vi "ReadnanoVNA.vi"() -> ()   [LabVIEW 2020]
panel:
  out "nanoVNA APP":T1
  out "string array 2":string[][](array[string])
  out "string array":string[](array[string])
  out "after substring":string
  out "text":string
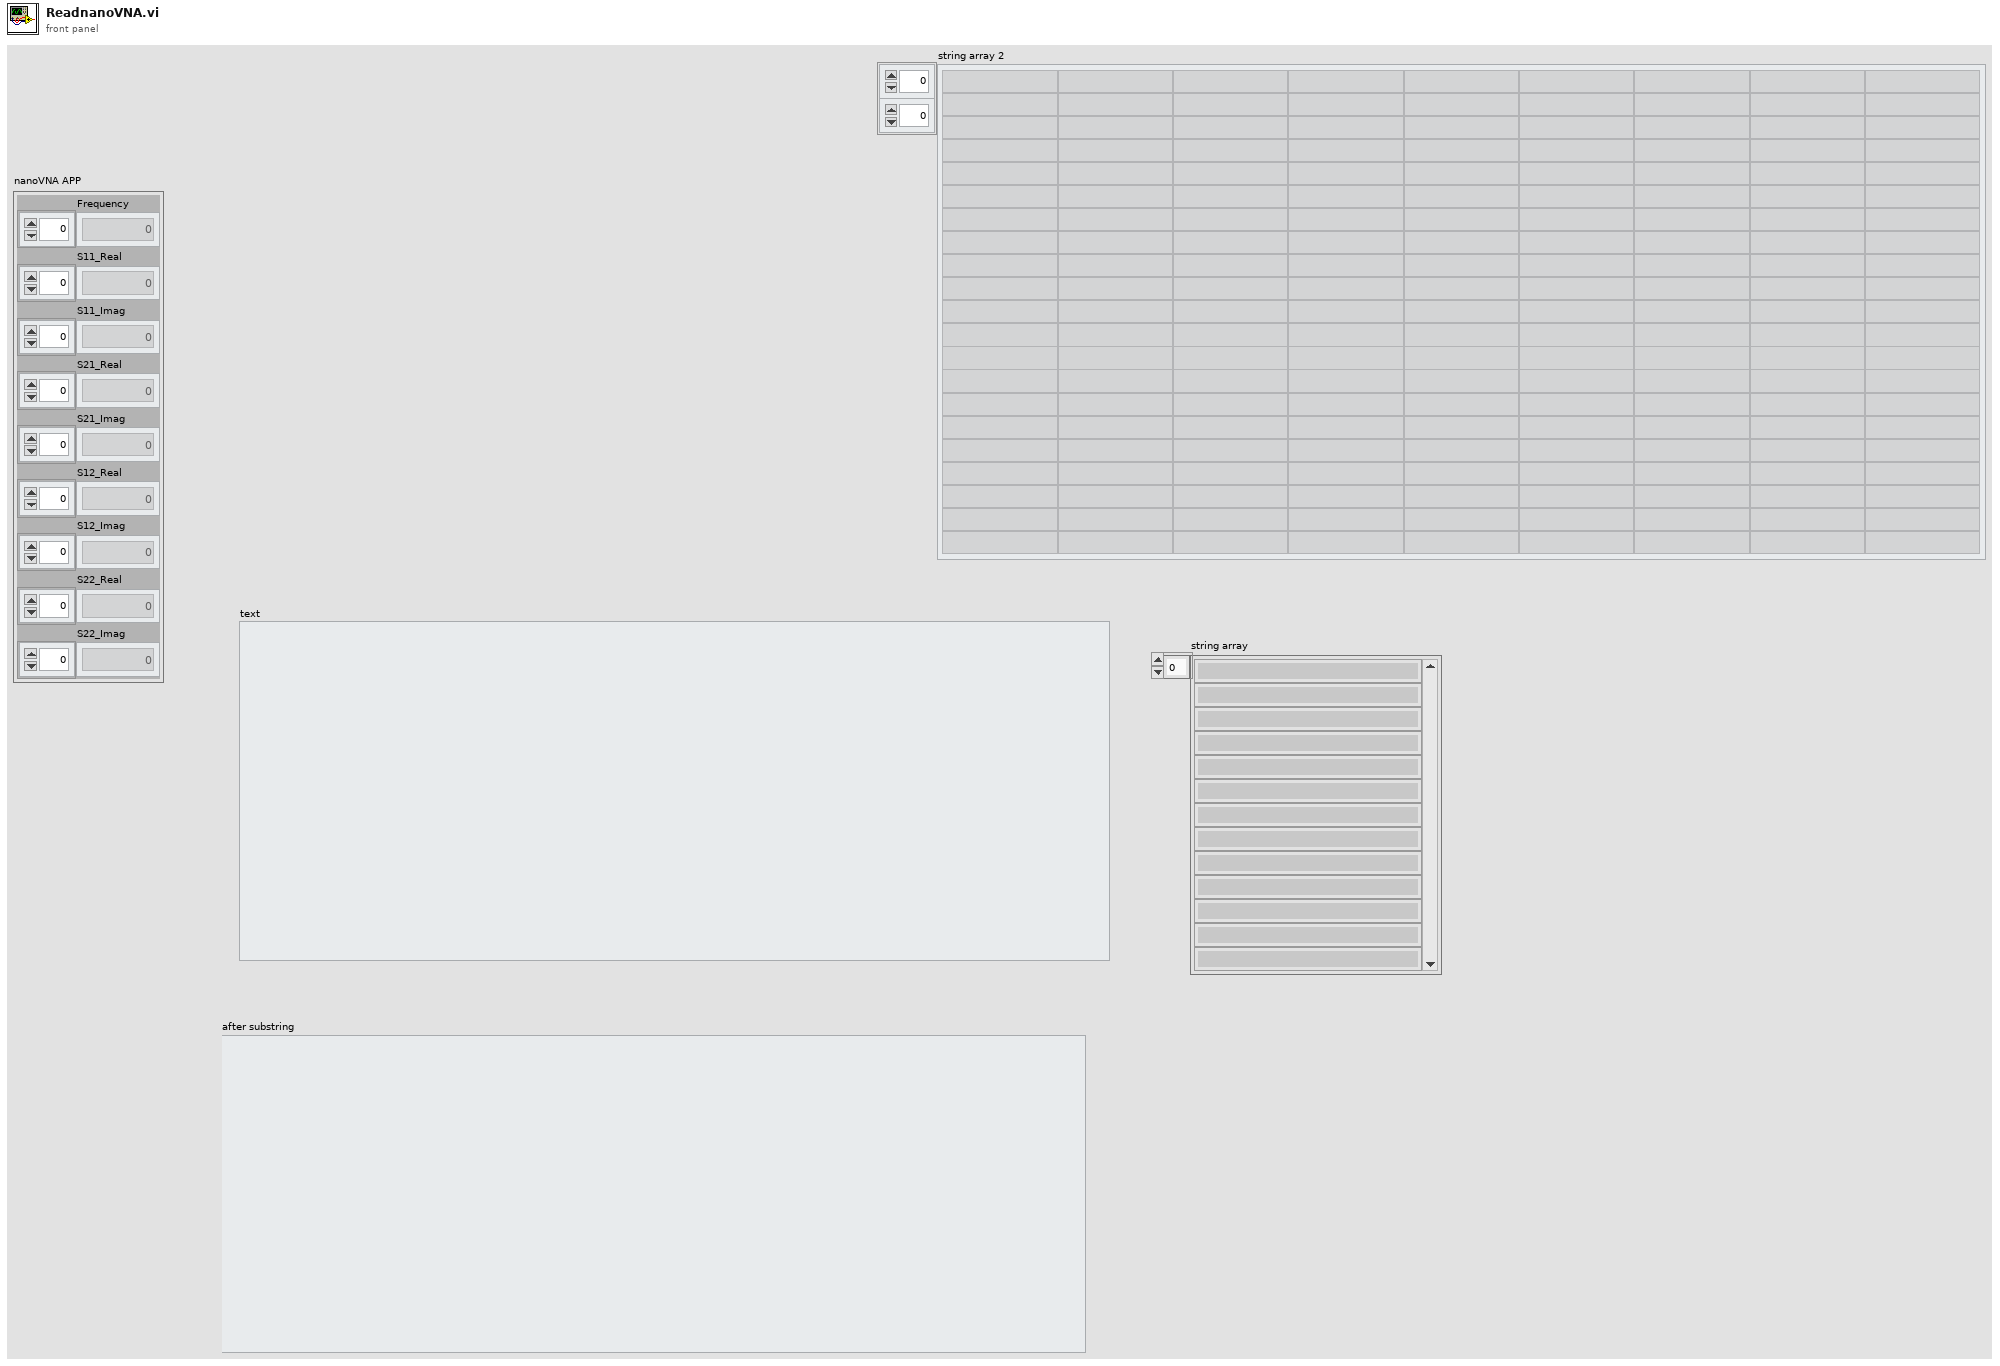
[diagram p1: front panel]
types:
  T1 = cluster{"Frequency":dbl[], "S11_Real":dbl[], "S11_Imag":dbl[], "S21_Real":dbl[], "S21_Imag":dbl[], "S12_Real":dbl[], "S12_Imag":dbl[], "S22_Real":dbl[], "S22_Imag":dbl[]}
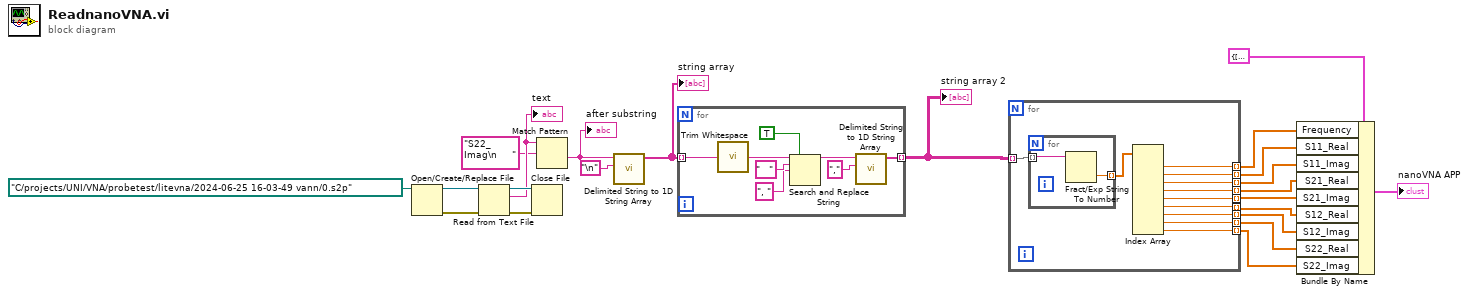
[diagram p0: block diagram]
diagram:
  n1 = Open/Create/Replace File(file path (use dialog)=path "C:/projects/UNI/VNA/probetest/litevna/2024-06-25 16-03-49 vann/0.s2p" ("file path (dialog if empty)")) -> (refnum out=w22:refnum<file>, error out=w19:errorcluster)  [unwired: 5 in, 1 out]
  n2 = Read from Text File(file (use dialog)=w22, error in=w19) -> (refnum out=w21:refnum<file>, text=w17:string, error out=w20:errorcluster)  [unwired: 2 in, 1 out]
  "text" <- w17
  n3 = Close File(refnum=w21, error in=w20) -> ()  [unwired: 2 out]
  n4 = Match Pattern(string=w17, regular expression="S22_Imag\n     " ("search string/char (-)")) -> (after substring=w13:string)  [unwired: 1 in, 3 out]
  "after substring" <- w13
  n5 = call <vilib>:"Delimited String to 1D String Array.vi"("delimiter"="\n", "delimited string"=w13) -> ("string array"=w14:string[])  [unwired: 9 in]
  "string array" <- w14
  n6 = for {
    tunnel: w14 -> [w30] mode=indexing
    tunnel: [w29] -> w12 mode=indexing
    n7 = call <vilib>:"Trim Whitespace.vi"("string"=w30) -> ("trimmed string"=w28:string)  [unwired: 1 in]
    n8 = Search and Replace String(replace all?=TRUE ("replace all? (F)"), input string=w28, search string="   ", replace string=", " ("replace string (\"\")")) -> (result string=w23:string)  [unwired: 4 in, 3 out]
    n9 = call <vilib>:"Delimited String to 1D String Array.vi"("delimiter"=",", "delimited string"=w23) -> ("string array"=w29:string[])  [unwired: 9 in]
  }
  "string array 2" <- w12
  n10 = for {
    tunnel: w12 -> [w41] mode=indexing
    tunnel: [w39] -> w9 mode=indexing
    tunnel: [w38] -> w8 mode=indexing
    tunnel: [w37] -> w7 mode=indexing
    tunnel: [w36] -> w6 mode=indexing
    tunnel: [w35] -> w5 mode=indexing
    tunnel: [w34] -> w4 mode=indexing
    tunnel: [w33] -> w3 mode=indexing
    tunnel: [w32] -> w2 mode=indexing
    tunnel: [w31] -> w1 mode=indexing
    n11 = for {
      tunnel: w41 -> [w43] mode=indexing
      tunnel: [w42] -> w40 mode=indexing
      n12 = Fract/Exp String To Number(string=w43) -> (number=w42:dbl)  [unwired: 3 in, 1 out]
    }
    n13 = Index Array(array=w40) -> (element #1=w39:dbl, element #2=w38:dbl, element #3=w37:dbl, element #4=w36:dbl, element #5=w35:dbl, element #6=w34:dbl, element #7=w33:dbl, element #8=w32:dbl, element #9=w31:dbl)  [unwired: 9 in]
  }
  n14 = Bundle By Name(cluster=T1 {"Frequency"=[], "S11_Real"=[], "S11_Imag"=[], "S21_Real"=[], "S21_Imag"=[], "S12_Real"=[], "S12_Imag"=[], "S22_Real"=[], "S22_Imag"=[]} ("nanoVNA APP"), "Frequency"=w9, "S11_Real"=w8, "S11_Imag"=w7, "S21_Real"=w6, "S21_Imag"=w5, "S12_Real"=w4, "S12_Imag"=w3, "S22_Real"=w2, "S22_Imag"=w1) -> (→"nanoVNA APP":T1)
